vi "LC Language Test.vi"() -> ()   [LabVIEW 2020]
doc: "sadasdsadasd"
panel:
  in  "选项卡控件":enum32{"选项卡 1", "选项卡 2"}(tab)
  in  "数组":T1(array[cluster])
  in  "按钮":bool
  out "波形图表":dbl(graph)
  in  "簇":cluster{"布尔":bool}
  in  "字符串":string
  in  "Botton04":bool caption="这是一个测试"
  in  "Test":bool caption="Triger"
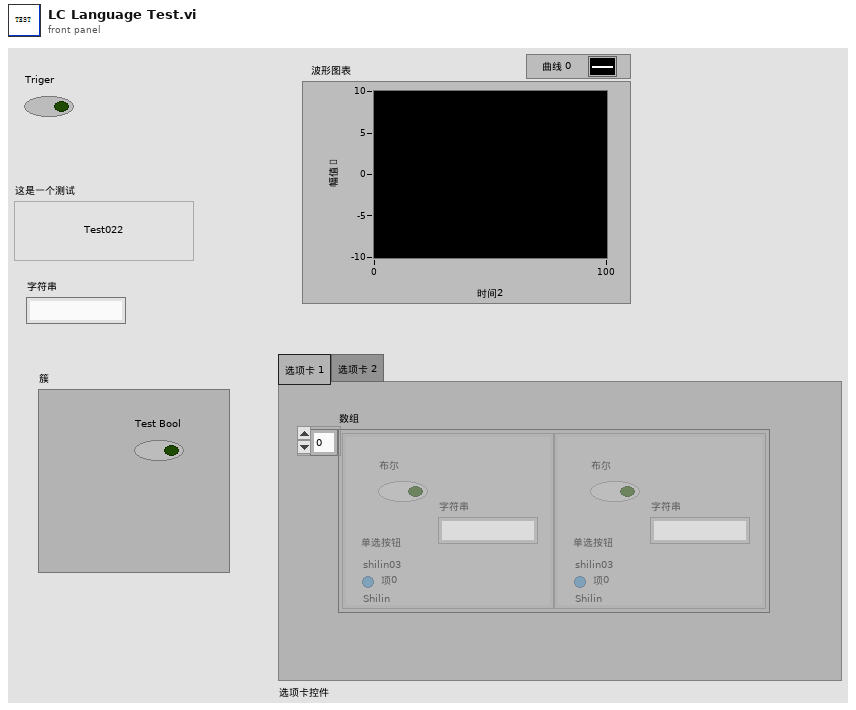
[diagram p1: front panel]
types:
  T1 = cluster{"布尔":bool, "字符串":string, "单选按钮":enum32{"Item 0", "Item 1"}}[]
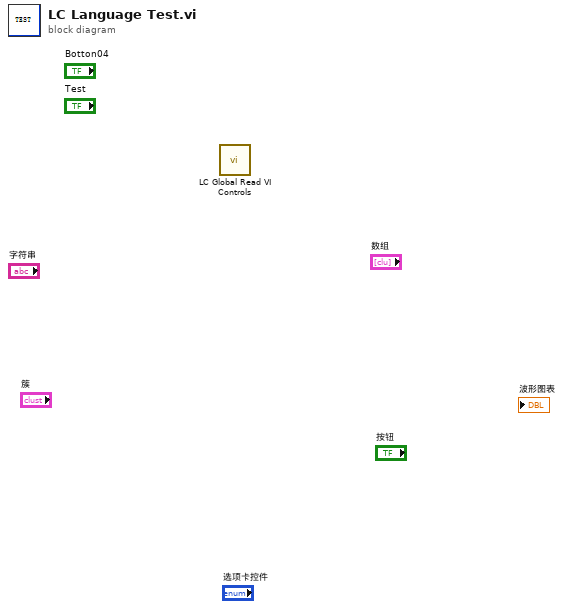
[diagram p0: block diagram]
diagram:
  n1 = call "LC Global Read VI Controls.vi"() -> ()  [unwired: 11 in, 1 out]
